vi "Check If Project Window Is Closed__icon_lib_labview_project_api.vi"(8 "error in (no error)":errorcluster, 11 "Project Reference":refnum<vi>) -> (0 "error out":errorcluster, 2 "Project Window Closed":bool, 3 "Project Reference Dup":refnum<vi>)   [LabVIEW 2016, in "LabVIEW Project API__icon_lib_labview_project_api.lvlib"]
doc: "Checks is Project Window is closed\n\n<b>Author:</b> JG\n\n<b>ICON Technologies Pty Ltd</b>\nCopyright (C) 1990-2009\nAll Rights Reserved"
uses:
  LabVIEW Project API__icon_lib_labview_project_api.lvlib
panel:
  # "Output"
  # "Input"
  # "ICON Technologies Pty Ltd\nCopyright (C) 1990-2009\nAll Rights Reserved"
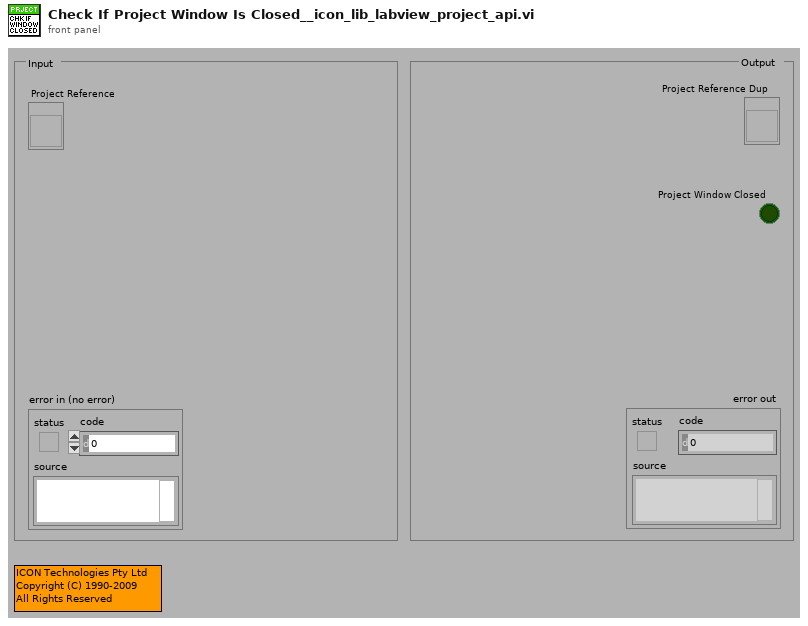
[diagram p1: front panel]
types:
  T1 = enum32{"Invalid", "Standard", "Closed", "Hidden", "Minimized", "Maximized"}
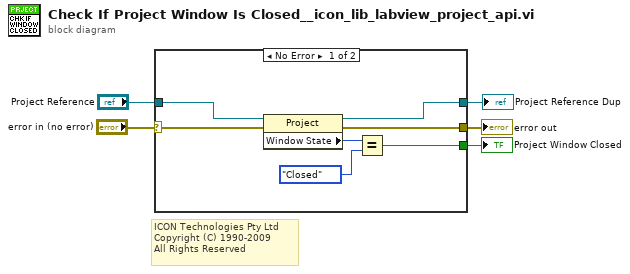
[diagram p0: block diagram]
diagram:
  # "ICON Technologies Pty Ltd\nCopyright (C) 1990-2009\nAll Rights Reserved"
  n1 = case shown="No Error" "error in (no error)" {
    selector: "error in (no error)" -> [w10 w14]
    tunnel: [w11 w14] -> w4
    tunnel: "Project Reference" -> [w12 w13]
    tunnel: [w9 w13] -> w2
    tunnel: [w8 _] -> w1
    frame No Error {
      n2 = property class="Project"(reference=w12, error in=w10) -> (reference out=w9:refnum<vi>, error out=w11:errorcluster, "Window State"=w7:T1)
      n3 = Equal?(x=w7, y=T1."Closed") -> (x = y?=w8:bool)
    }
    frame Error {
    }
  }
  "error out" <- w4
  "Project Reference Dup" <- w2
  "Project Window Closed" <- w1
